vi "Property Nodes - Fill Tank Color.vi"() -> ()   [LabVIEW 2012]
panel:
  in  "停止按钮":bool
  out "液罐":dbl(slide) scale=0.0..10.0
  in  "警告等级":dbl(slide) scale=0.0..10.0
  in  "填充等级":dbl(slide) scale=0.0..10.0
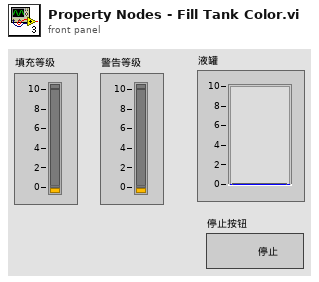
[diagram p1: front panel]
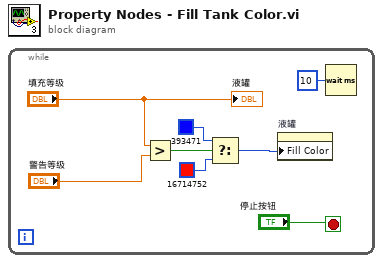
[diagram p0: block diagram]
diagram:
  n1 = while {
    stop <- "停止按钮" stop-if-true
    n2 = Greater? ("大于？")(x="填充等级", y="警告等级") -> (0:w3:bool)
    n3 = Select ("选择")(t=u32 393471, s=w3, f=u32 16714752) -> (s? t:f=w1:u32)
    n4 = property on="液罐" class="Slide (严格)"("Fill Color"=w1) -> ()  [unwired: 2 in, 2 out]
    n5 = Wait (ms) ("等待(ms)")(milliseconds to wait=u32 10 ("等待时间（毫秒）")) -> ()  [unwired: 1 out]
    "液罐" <- "填充等级"
  }
